vi "HGF_SVVisitor_deregister.appendData2Variant.vi"(0 "variant":variant, 1 "Shared Variable Control (DSC)":refnum<k21>, 2 "HGF_NetworkVisitor":refnum<class "HGF_NetworkVisitor.lvclass">, 3 "HGF_TriggeredEvent":refnum<class "HGF_TriggeredEvent.lvclass">, 4 "shared variable refnum (without DSC)":refnum<k21>, 5 "error in":errorcluster, 7 "Rem SV/Visitor from List":bool) -> (14 "dup variant":variant, 19 "error out":errorcluster)   [LabVIEW 2012, in "HGF_SV.lvlib" / "HGF_SVMonitorVisitor_deregister.lvclass"]
uses:
  HGF_SVMonitorVisitor_deregister.lvclass
  HGF_BaseClasses/HGF_NetworkVisitor/HGF_NetworkVisitor.lvclass
  HGF_BaseClasses/HGF_TriggeredEvent/HGF_TriggeredEvent.lvclass
  <resource>/objmgr/ni.var.rc
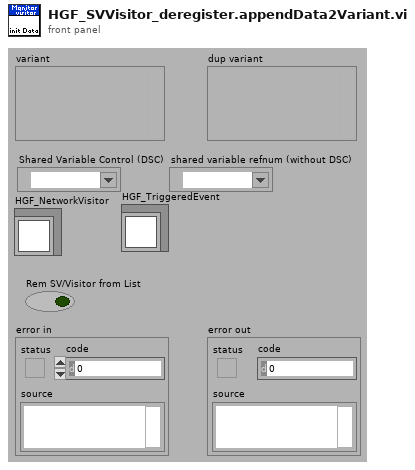
[diagram p1: front panel]
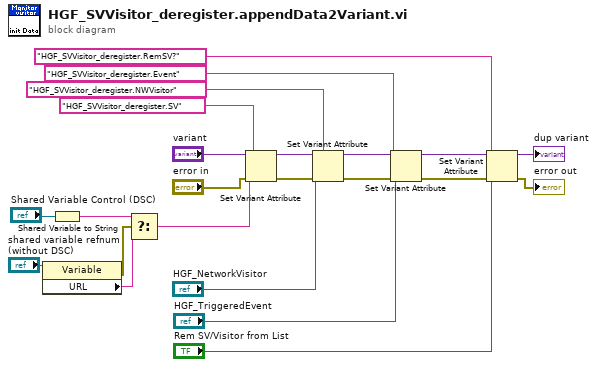
[diagram p0: block diagram]
diagram:
  n1 = property class="Variable"(reference="shared variable refnum (without DSC)") -> (error out=w1:errorcluster, "URL"=w6:string)  [unwired: 1 in, 1 out]
  n2 = Shared Variable to String(1:"Shared Variable Control (DSC)") -> (0:w5:string)
  n3 = Select(t=w5, s=w1, f=w6) -> (s? t:f=w2:string)
  n4 = Set Variant Attribute(Variant="variant", name="HGF_SVVisitor_deregister.SV", value=w2, error in="error in") -> (Variant out=w11:variant, error out=w22:errorcluster)  [unwired: 1 out]
  n5 = Set Variant Attribute(Variant=w11, name="HGF_SVVisitor_deregister.NWVisitor", value="HGF_NetworkVisitor", error in=w22) -> (Variant out=w12:variant, error out=w21:errorcluster)  [unwired: 1 out]
  n6 = Set Variant Attribute(Variant=w12, name="HGF_SVVisitor_deregister.Event", value="HGF_TriggeredEvent", error in=w21) -> (Variant out=w13:variant, error out=w20:errorcluster)  [unwired: 1 out]
  n7 = Set Variant Attribute(Variant=w13, name="HGF_SVVisitor_deregister.RemSV?", value="Rem SV/Visitor from List", error in=w20) -> (Variant out=→"dup variant":variant, error out=→"error out":errorcluster)  [unwired: 1 out]
